vi "DropDetection NaamaVision.vi"(7 "Frame Number":u32, 8 "error in":errorcluster, 9 "Image in":T1(plugin-control), 10 "Minimum Match Score":sgl=400.0, 11 "Path":path=path "Z:/Downloads/Fridge Pictures/1") -> (0 "error out":errorcluster, 1 "Number of Matches":i32, 2 "Matches (pixel)":T2(array[cluster]), 3 "Image Out":T1(plugin-control))   [LabVIEW 2013]
uses:
  <vilib>/vision/NI_Vision_Development_Module.lvlib
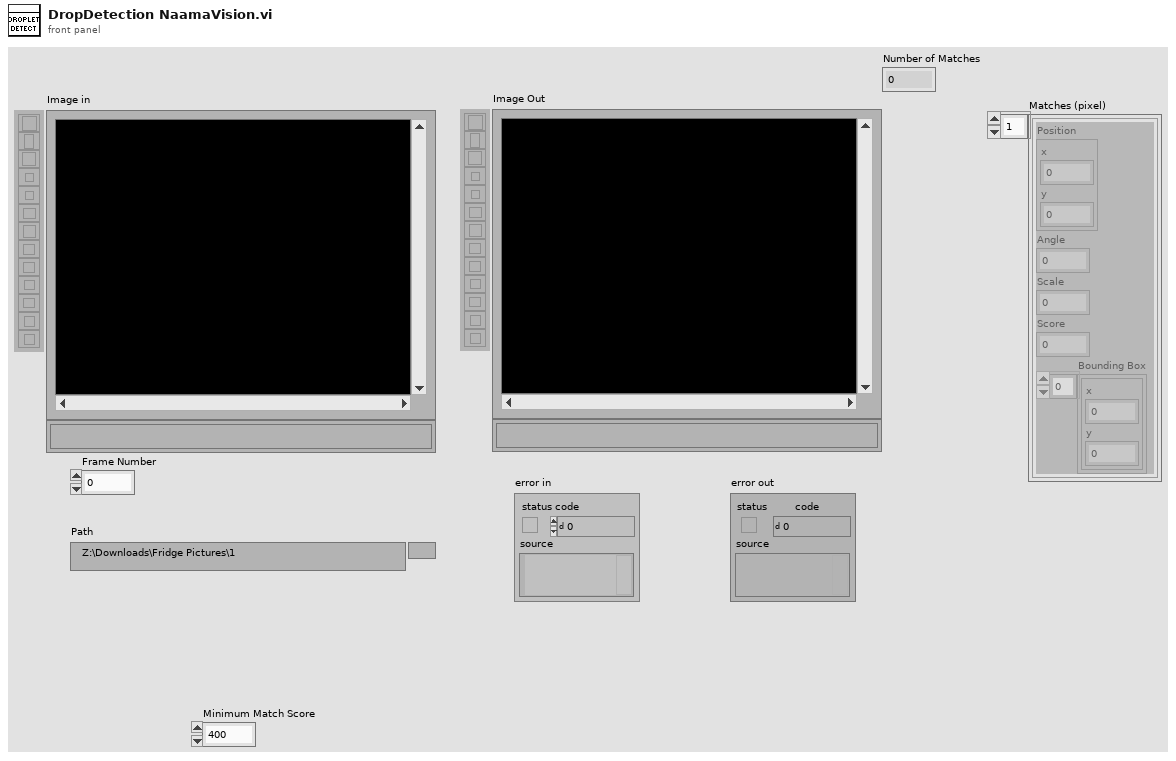
[diagram p1: front panel]
types:
  T1 = typedef "IMAQ Image.ctl" = refnum<image>
  T2 = cluster{"Position":cluster{"x":sgl, "y":sgl}, "Angle":sgl, "Scale":sgl, "Score":sgl, "Bounding Box":cluster{"x":sgl, "y":sgl}[]}[]
  T3 = cluster{"Global Rectangle":i32[], "Contours":cluster{"ID":enum32{"External", "Internal"}, "Type":u32, "Coordinates":i32[]}[]}
  T4 = typedef "IMAQ AVI2 Refnum.ctl" = refnum<k20>
  T5 = cluster{"Number of Matches Requested":i32, "Minimum Match Score":sgl, "Angle Ranges":cluster{"Start Angle":sgl, "End Angle":sgl}[]}
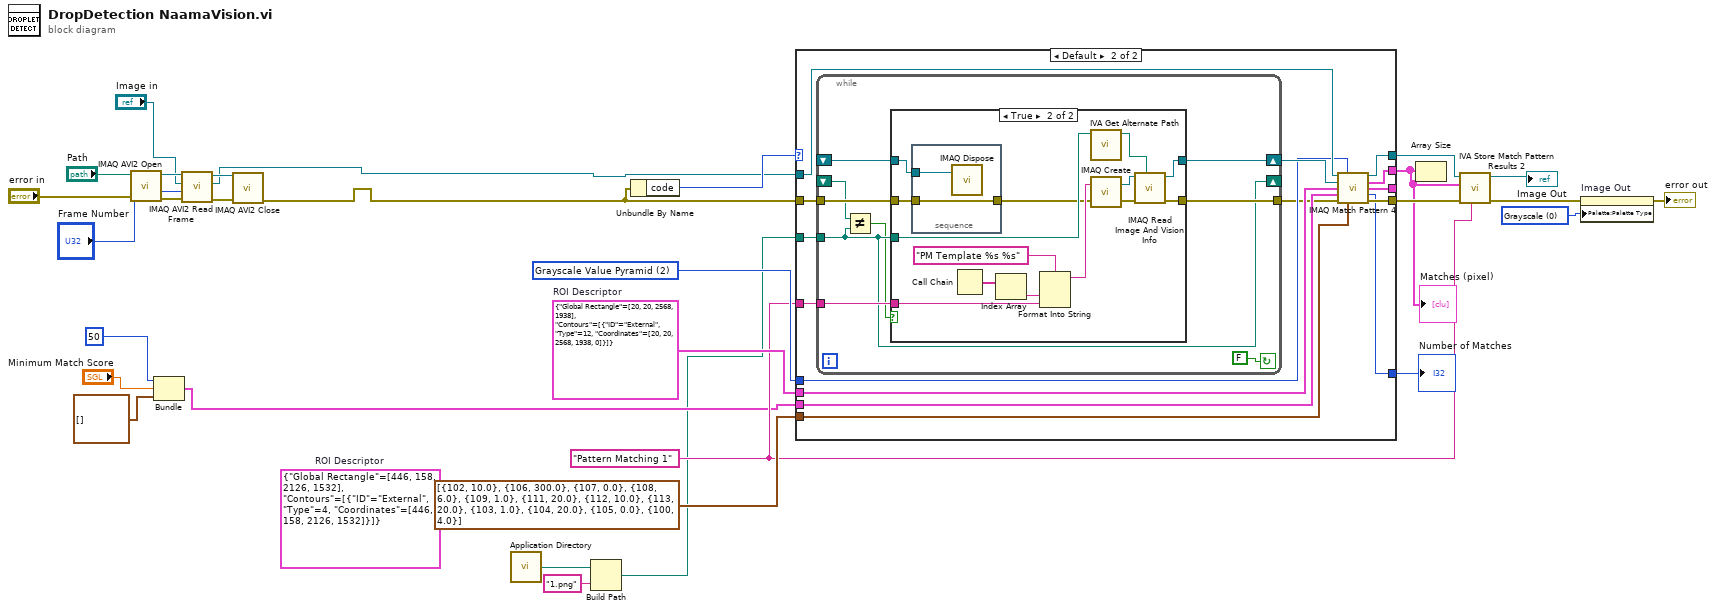
[diagram p0: block diagram]
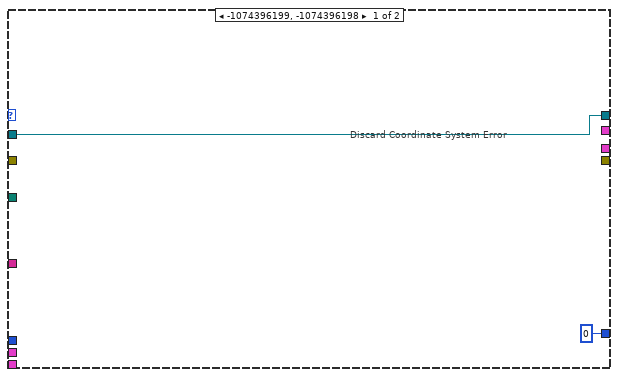
[diagram p2: hidden frame]
diagram:
  w22 = u32 0 items=["Grayscale", "Binary", "Gradient", "Rainbow", "Temperature", "User Defined"] ("Palette")
  w27 = 2 items=["All", "Low Discrepancy Sampling", "Grayscale Value Pyramid", "Gradients Pyramid"] ("Algorithm")
  w24 = "Pattern Matching 1" ("Step Name")
  w26 = T3 {"Global Rectangle"=[20, 20, 2568, 1938], "Contours"=[{"ID"=enum."External", "Type"=12, "Coordinates"=[20, 20, 2568, 1938, 0]}]}  # ROI Descriptor
  (unwired) T3 {"Global Rectangle"=[446, 158, 2126, 1532], "Contours"=[{"ID"=enum."External", "Type"=4, "Coordinates"=[446, 158, 2126, 1532]}]}  # ROI Descriptor
  n1 = call "IMAQ AVI2 Open"("error in (no error)"="error in", "AVI File Path"="Path") -> ("error out"=w9:errorcluster, "AVI Refnum"=w8:T4)  [unwired: 8 in]
  n2 = Bundle("Number of Matches Requested"=50, "Minimum Match Score"="Minimum Match Score", "Angle Ranges"=cluster{"Start Angle":sgl, "End Angle":sgl}[] []) -> (w14:T5)  [unwired: 1 in]
  n3 = call "IMAQ AVI2 Read Frame"("error in (no error)"=w9, "Frame Number"="Frame Number", "Image"="Image in", "AVI Refnum"=w8) -> ("error out"=w4:errorcluster, "Image Out"=w2:T1, "AVI Refnum (duplicate)"=w3:T4)  [unwired: 5 in]
  n4 = call "IMAQ AVI2 Close"("error in (no error)"=w4, "AVI Refnum"=w3) -> ("error out"=w1:errorcluster)  [unwired: 9 in]
  n5 = call <vilib>:"Application Directory.vi"() -> ("Application Directory"=w13:path)
  n6 = Build Path(base path=w13, name or relative path="1.png") -> (appended path=w11:path)
  n7 = Unbundle By Name(w1) -> ("code"=w28:i32)
  n8 = case shown="Default" w28 {
    tunnel: w11 -> [_ w47]
    tunnel: w1 -> [_ w46]
    tunnel: w2 -> [w32 w41]
    tunnel: [_ w42] -> w30
    tunnel: [_ w43] -> w23
    tunnel: [w32 w40] -> w29
    tunnel: w24 -> [_ w45]
    tunnel: w27 -> [_ w39]
    tunnel: w26 -> [_ w38]
    tunnel: w14 -> [_ w37]
    tunnel: cluster{"Item":u16, "Value":dbl}[] [{"Item"=102, "Value"=10.0}, {"Item"=106, "Value"=300.0}, {"Item"=107, "Value"=0.0}, {"Item"=108, "Value"=6.0}, {"Item"=109, "Value"=1.0}, {"Item"=111, "Value"=20.0}, {"Item"=112, "Value"=10.0}, {"Item"=113, "Value"=20.0}, {"Item"=103, "Value"=1.0}, {"Item"=104, "Value"=20.0}, {"Item"=105, "Value"=0.0}, {"Item"=100, "Value"=4.0}] ("Advanced Options") -> [_ w35]
    tunnel: [_ w34] -> _
    tunnel: [0 ("Number of Matches") w33] -> w19
    frame -1074396199, -1074396198 {
      # "Discard Coordinate System Error"
    }
    frame Default {
      n9 = while {
        shift-right: [w56] -> w44
        shift-left: _ -> [w55]
        tunnel: [w53] -> w36
        tunnel: w46 -> [w52]
        tunnel: w47 -> [w49]
        tunnel: w45 -> [w51]
        shift-right: [w49] -> _
        shift-left: _ -> [w50]
        stop <- FALSE continue-if-true
        n10 = Not Equal?(x=w50, y=w49) -> (x != y?=w48:bool)
        n11 = case shown="True" w48 {
          tunnel: [w58 w70] -> w56
          tunnel: w55 -> [w58 w61]
          tunnel: [w57 w67] -> w53
          tunnel: w52 -> [w57 w60]
          tunnel: w49 -> [_ w63]
          tunnel: w51 -> [_ w64]
          frame False {
          }
          frame True {
            n12 = stacked-sequence {
              tunnel: w61 -> [w74]
              tunnel: w60 -> [w73]
              tunnel: [w73] -> w59
              frame #0 {
                n13 = call "IMAQ Dispose"("Image"=w74) -> ()  [unwired: 2 in, 4 out]
              }
            }
            n14 = Call Chain() -> (call chain=w66:string[])
            n15 = Index Array(array=w66) -> (element=w65:string)  [unwired: 1 in]
            n16 = Format Into String(format string="PM Template %s %s" ("Image Name"), w65, w64) -> (resulting string=w72:string)  [unwired: 2 in, 1 out]
            n17 = call <vilib>:"IVA Get Alternate Path.vi"("Path In"=w63) -> ("Path Out"=w62:path)  [unwired: 10 out]
            n18 = call "IMAQ Create"("Image Name"=w72, "error in (no error)"=w59) -> ("New Image"=w69:T1, "error out"=w68:errorcluster)  [unwired: 2 in, 1 out]
            n19 = call "IMAQ Read Image And Vision Info"("File Path"=w62, "error in (no error)"=w68, "Image"=w69) -> ("error out"=w67:errorcluster, "Image Out"=w70:T1)  [unwired: 1 in, 6 out]
          }
        }
      }
      n20 = call "IMAQ Match Pattern 4"("Image"=w41, "Algorithm"=w39, "Template Image"=w44, "ROI Descriptor"=w38, "Parameters"=w37, "error in (no error)"=w36, "Advanced Options"=w35) -> ("Image (duplicate)"=w40:T1, "Matches (pixel)"=w43:T2, "Matches (real-world)"=w34:T2, "Number of Matches"=w33:i32, "error out"=w42:errorcluster)  [unwired: 4 in]
    }
  }
  "Matches (pixel)" <- w23
  "Number of Matches" <- w19
  n21 = Array Size(array=w23) -> ()  [unwired: 1 out]
  n22 = call <vilib>:"IVA Store Match Pattern Results 2.vi"("Step Name"=w24, "error in (no error)"=w30, "Matches (pixel)"=w23, "Image in"=w29) -> ("error out"=w21:errorcluster, "Image dup"=→"Image Out":T1)  [unwired: 2 in, 4 out]
  n23 = property on="Image Out" class="ImageControl"(error in=w21, "Palette:Palette Type"=w22) -> (error out=→"error out":errorcluster)  [unwired: 1 in, 1 out]
